vi "NIN3D Coordinate Conversion.vi"(0 "X":sgl, 1 "Z_prev":sgl, 2 "Y_prev":sgl, 3 "X_prev":sgl, 5 "Y":sgl, 7 "Z":sgl, 11 "Coordinate System":enum16{"Cartesian", "Cylindrical", "Spherical"}(ring)) -> (4 "X out":sgl, 6 "Y out":sgl, 8 "Z out":sgl, 15 "NaN?":bool)   [LabVIEW 2020]
uses:
  <vilib>/Analysis/NI_AALPro.lvlib
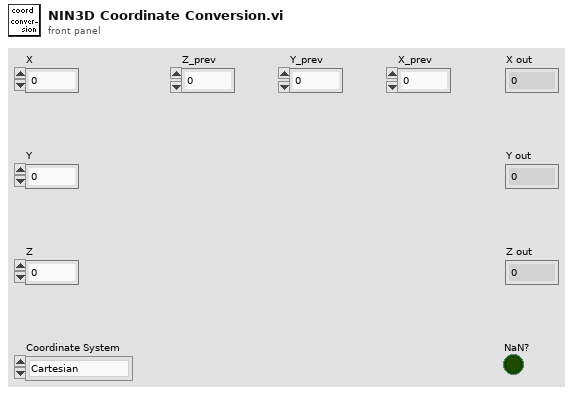
[diagram p1: front panel]
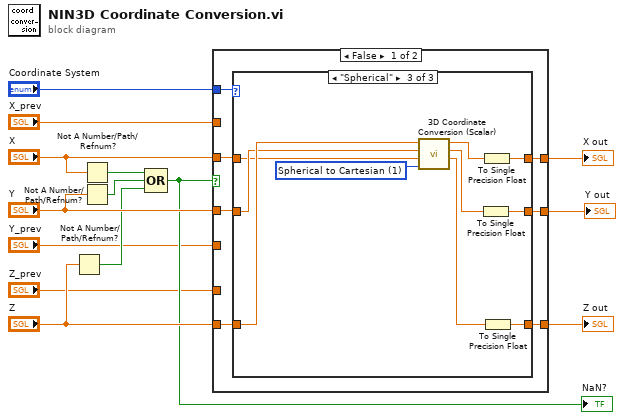
[diagram p0: block diagram]
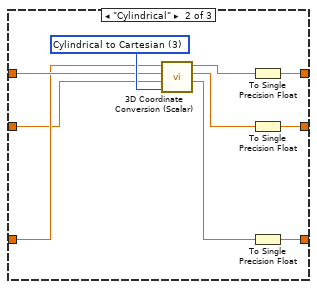
[diagram p3: hidden frame]
diagram:
  n1 = Not A Number/Path/Refnum?(number/path/refnum="Z") -> (NaN/Path/Refnum?=w4:bool)
  n2 = Not A Number/Path/Refnum?(number/path/refnum="X") -> (NaN/Path/Refnum?=w6:bool)
  n3 = Not A Number/Path/Refnum?(number/path/refnum="Y") -> (NaN/Path/Refnum?=w5:bool)
  n4 = Compound Arithmetic op=OR(w6, w5, w4) -> (w7:bool)
  "NaN?" <- w7
  n5 = case shown="False" w7 {
    tunnel: [w21 w46] -> w14
    tunnel: [w20 w45] -> w13
    tunnel: "Coordinate System" -> [w19 _]
    tunnel: [w18 w47] -> w11
    tunnel: "X" -> [w17 _]
    tunnel: "Y" -> [w16 _]
    tunnel: "Z" -> [w15 _]
    tunnel: "X_prev" -> [_ w47]
    tunnel: "Y_prev" -> [_ w46]
    tunnel: "Z_prev" -> [_ w45]
    frame False {
      n6 = case shown="\"Spherical\"" w19 {
        tunnel: w17 -> [w24 w33 w38]
        tunnel: w15 -> [w22 w32 w44]
        tunnel: w16 -> [w23 w31 w39]
        tunnel: [w24 w27 w37] -> w18
        tunnel: [w23 w26 w36] -> w21
        tunnel: [w22 w25 w35] -> w20
        frame "Cartesian", Default {
        }
        frame "Cylindrical" {
          w34 = u16 3 items=["Cartesian to Spherical", "Spherical to Cartesian", "Cartesian to Cylindrical", "Cylindrical to Cartesian", "Spherical to Cylindrical", "Cylindrical to Spherical"] ("conversion type")
          n7 = call <vilib>:"3D Coordinate Conversion (Scalar).vi"("conversion type"=w34, "axis 3"=w31, "axis 2"=w33, "axis 1"=w32) -> ("axis 3 out"=w28:dbl, "axis 2 out"=w29:dbl, "axis 1 out"=w30:dbl)  [unwired: 5 out]
          n8 = To Single Precision Float(number=w30) -> (single precision float=w27:sgl)
          n9 = To Single Precision Float(number=w29) -> (single precision float=w26:sgl)
          n10 = To Single Precision Float(number=w28) -> (single precision float=w25:sgl)
        }
        frame "Spherical" {
          w40 = u16 1 items=["Cartesian to Spherical", "Spherical to Cartesian", "Cartesian to Cylindrical", "Cylindrical to Cartesian", "Spherical to Cylindrical", "Cylindrical to Spherical"] ("conversion type")
          n11 = call <vilib>:"3D Coordinate Conversion (Scalar).vi"("conversion type"=w40, "axis 3"=w38, "axis 2"=w39, "axis 1"=w44) -> ("axis 3 out"=w41:dbl, "axis 2 out"=w42:dbl, "axis 1 out"=w43:dbl)  [unwired: 5 out]
          n12 = To Single Precision Float(number=w42) -> (single precision float=w36:sgl)
          n13 = To Single Precision Float(number=w43) -> (single precision float=w37:sgl)
          n14 = To Single Precision Float(number=w41) -> (single precision float=w35:sgl)
        }
      }
    }
    frame True {
    }
  }
  "X out" <- w11
  "Y out" <- w14
  "Z out" <- w13
